vi "Generate 16ms Pulse and Get ADC Volts.vi"(0 "Channel names":string="Dev1/ao0", 1 "offset":dbl=2.25, 3 "#Samples":i32=1000, 5 "rate":dbl=1000.0, 7 "nWhichChan":i32, 9 "frequency":dbl=62.5, 11 "error in":errorcluster, 12 "square wave \nduty cycle (%)":dbl=50.0, 13 "nScale":i32=2, 14 "amplitude (pk)":dbl=5.0) -> (4 "task out":refnum<k21>, 6 "Channel Voltage Result":dbl, 15 "error out":errorcluster)   [LabVIEW 2013]
doc: "This VI generates the square wave and use the ReadChanValue dll function call to get ADC volts"
uses:
  <vilib>/DAQmx/write.llb/DAQmx Write (Analog 1D Wfm NChan NSamp).vi
  <vilib>/DAQmx/create/channels.llb/DAQmx Create Channel (AO-Voltage-Basic).vi
  <vilib>/DAQmx/configure/timing.llb/DAQmx Timing (Sample Clock).vi
  <vilib>/DAQmx/miscellaneous.llb/DAQmx Fill In Error Info.vi
  <resource>/objmgr/daqmx.rc
  <vilib>/measure/NI_MABase.lvlib
panel:
  out "Waveform Graph":waveform(dbl)(graph)={"t0"=timestamp(0 s since 1904-01-01), "dt"=2e-05, "Y"=array[5000 elements]}
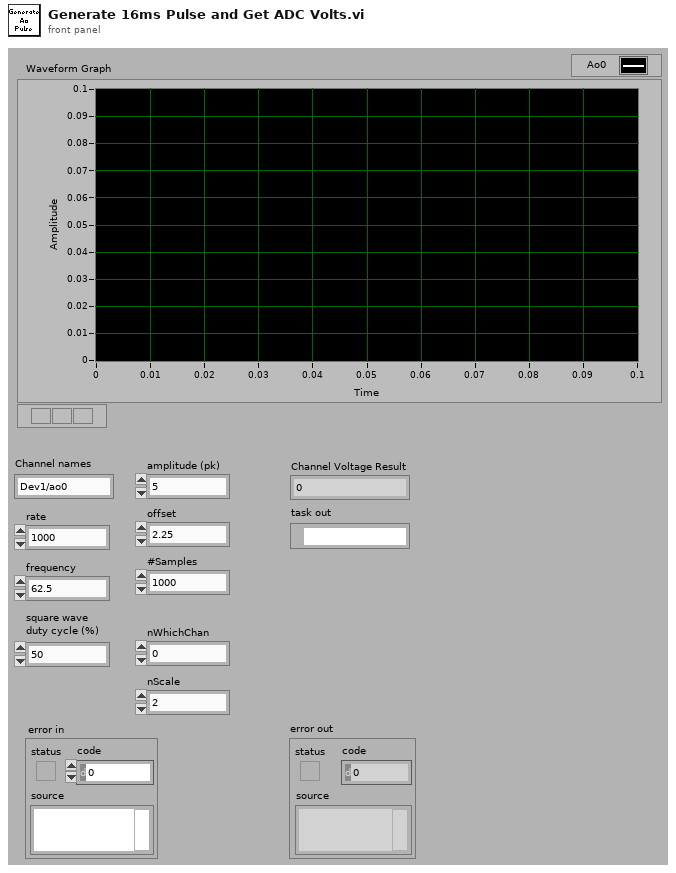
[diagram p1: front panel]
types:
  T1 = enum16{"Sine Wave", "Triangle Wave", "Square Wave", "Sawtooth Wave"}
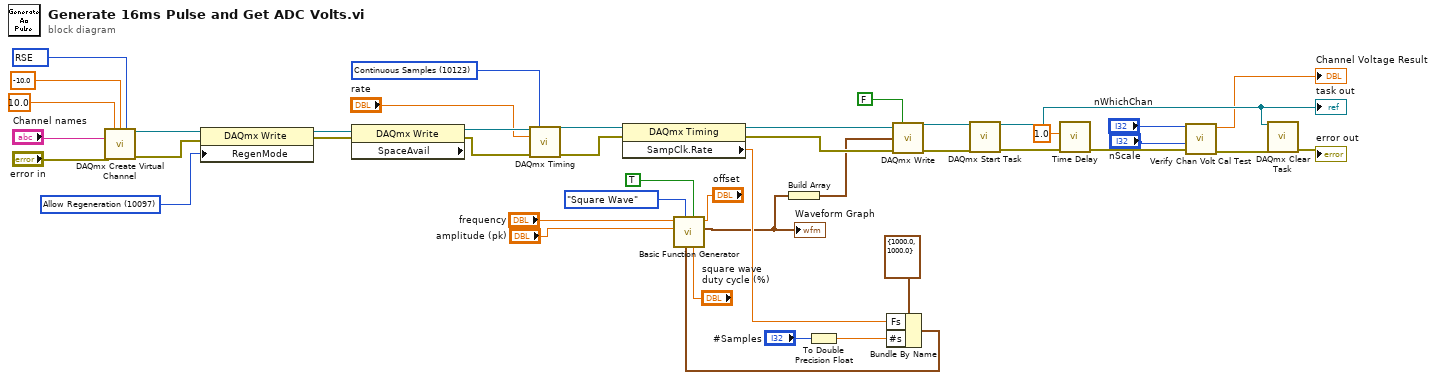
[diagram p0: block diagram]
diagram:
  w10 = 10123 items=["Finite Samples"=10178, "Continuous Samples"=10123, "Hardware Timed Single Point"=12522] ("sample mode")
  w13 = 10083 items=["Default"=-1, "RSE"=10083, "Differential"=10106, "Pseudodifferential"=12529] ("output terminal configuration")
  w41 = 10097 items=["Allow Regeneration"=10097, "Do Not Allow Regeneration"=10158] ("RegenMode")
  n1 = call-poly <vilib>:"DAQmx Create Virtual Channel.vi"("maximum value"=10.0, "minimum value"=-10.0, "output terminal configuration"=w13, "physical channels"="Channel names", "error in"="error in") -> ("task out"=w43:refnum<k21>, "error out"=w42:errorcluster)  [unwired: 9 in]
  n2 = property class="DAQmx Write"(reference=w43, error in=w42, "RegenMode"=w41) -> (reference out=w39:refnum<k21>, error out=w40:errorcluster)
  n3 = property class="DAQmx Write" props=["SpaceAvail"](reference=w39, error in=w40) -> (reference out=w38:refnum<k21>, error out=w37:errorcluster)  [unwired: 1 out]
  n4 = call-poly <vilib>:"DAQmx Timing.vi"("task/channels in"=w38, "sample mode"=w10, "rate"="rate", "error in"=w37) -> ("task out"=w36:refnum<k21>, "error out"=w35:errorcluster)  [unwired: 10 in]
  n5 = property class="DAQmx Timing"(reference=w36, error in=w35) -> (reference out=w18:refnum<k21>, error out=w19:errorcluster, "SampClk.Rate"=w29:dbl)
  n6 = To Double Precision Float(number="#Samples") -> (double precision float=w28:dbl)
  n7 = Bundle By Name(cluster=cluster{"Fs":dbl, "#s":dbl} {"Fs"=1000.0, "#s"=1000.0} ("sampling info"), "Fs"=w29, "#s"=w28) -> (w31:cluster{"Fs":dbl, "#s":dbl})
  n8 = call <vilib>:"Basic Function Generator.vi"("offset"="offset", "square wave duty cycle (%)"="square wave \nduty cycle (%)", "reset signal"=TRUE, "sampling info"=w31, "signal type"=T1."Square Wave", "amplitude"="amplitude (pk)", "frequency"="frequency") -> ("signal out"=w11:waveform(dbl))  [unwired: 2 in, 2 out]
  "Waveform Graph" <- w11
  n9 = Build Array(w11) -> (w12:waveform(dbl)[])
  n10 = call-poly <vilib>:"DAQmx Write.vi"("task/channels in"=w18, "auto start"=FALSE, "data"=w12, "error in"=w19) -> ("task out"=w16:refnum<k21>, "error out"=w17:errorcluster)  [unwired: 9 in, 1 out]
  n11 = call <vilib>:"DAQmx Start Task.vi"("task/channels in"=w16, "error in"=w17) -> ("task out"=w9:refnum<k21>, "error out"=w6:errorcluster)  [unwired: 12 in]
  "task out" <- w9
  n12 = call "Time Delay"("error in (no error)"=w6, "Delay Time (s)"=1.0) -> ("error out"=w5:errorcluster)  [unwired: 9 in]
  n13 = call "Verify Chan Volt Cal Test.vi"("error in (no error)"=w5, "nScale"="nScale", "nWhichChan"="nWhichChan") -> ("error out"=w7:errorcluster, "Channel Voltage Result"=→"Channel Voltage Result":dbl)  [unwired: 7 in]
  n14 = call <vilib>:"DAQmx Clear Task.vi"("task in"=w9, "error in"=w7) -> ("error out"=→"error out":errorcluster)  [unwired: 13 in]
